vi "Command_Passive_Flywheel.vi"(0 "Startup":bool, 2 "Timeout":dbl, 3 "RPM":dbl) -> (6 "Reint":bool, 7 "Completed":bool, 9 "Output_RPM":dbl)   [LabVIEW 2020]
uses:
  Auto Utilities/Command_Execution_State.ctl
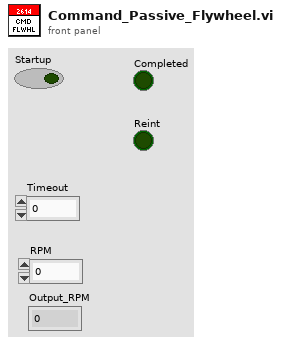
[diagram p1: front panel]
types:
  T1 = typedef "Command_Execution_State.ctl" = enum16{"Initialize", "Execute", "Finish"}
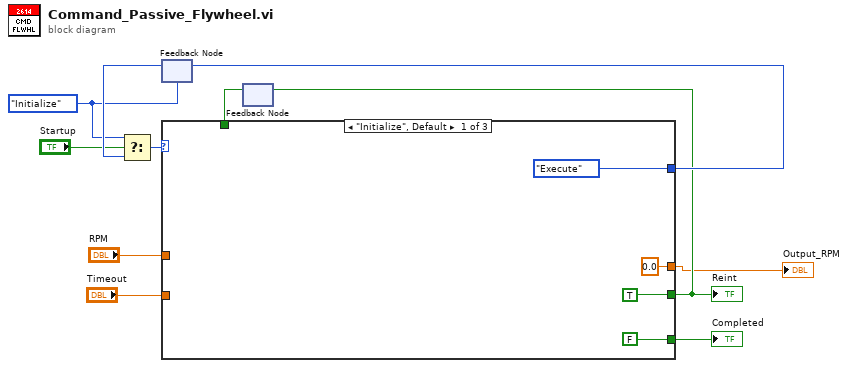
[diagram p0: block diagram]
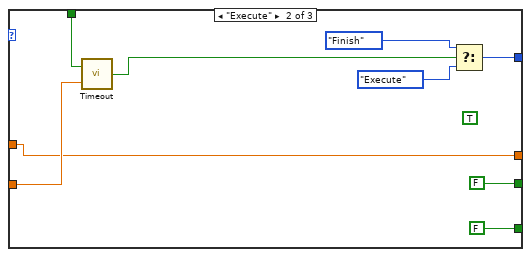
[diagram p2: hidden frame]
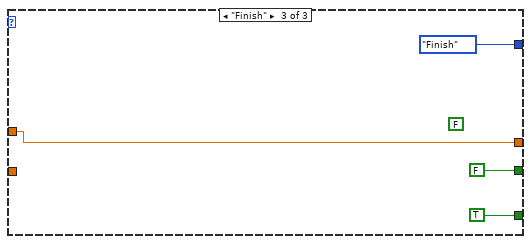
[diagram p3: hidden frame]
diagram:
  w6 = Command_Execution_State."Initialize" ("Play State")
  n1 = feedback #1(w6) -> (w9:T1)
  n2 = Select(t=w6, s="Startup", f=w9) -> (s? t:f=w11:T1)
  n3 = feedback #2() -> (w5:bool)  [unwired: 1 in]
  n4 = case shown="\"Initialize\", Default" w11 {
    tunnel: [Command_Execution_State."Execute" ("Play State") w20 Command_Execution_State."Finish" ("Play State")] -> w10
    tunnel: [FALSE FALSE TRUE] -> w8
    tunnel: [TRUE FALSE FALSE] -> w3
    tunnel: w5 -> [_ w22 _]
    tunnel: "Timeout" -> [_ w21 _]
    tunnel: "RPM" -> [_ w16 w25]
    tunnel: [0.0 ("RPM") w16 w25] -> w1
    frame "Initialize", Default {
    }
    frame "Execute" {
      (unwired) TRUE
      n5 = call "Timeout.vi"("Timeout"=w21, "Initialize"=w22) -> ("Timed Out?"=w17:bool)
      n6 = Select(t=Command_Execution_State."Finish" ("Play State"), s=w17, f=Command_Execution_State."Execute" ("Play State")) -> (s? t:f=w20:T1)
    }
    frame "Finish" {
      (unwired) FALSE
    }
  }
  "Completed" <- w8
  "Reint" <- w3
  "Output_RPM" <- w1
  n7 = feedback-in #1(w10) -> ()
  n8 = feedback-in #2(w3) -> ()
